vi "AllShipsSunk.vi"(0 "object in":refnum<class "Map.lvclass">, 5 "error in (no error)":errorcluster) -> (14 "object out":refnum<class "Map.lvclass">, 16 "AllShipsSunk?":bool, 19 "error out":errorcluster)   [LabVIEW 2015, in "Map.lvclass"]
doc: "Returns true if all ships on the map are sunk."
uses:
  Map.lvclass
  Map.lvclass/Map.ctl
  Battleship_class/Battleship.lvclass
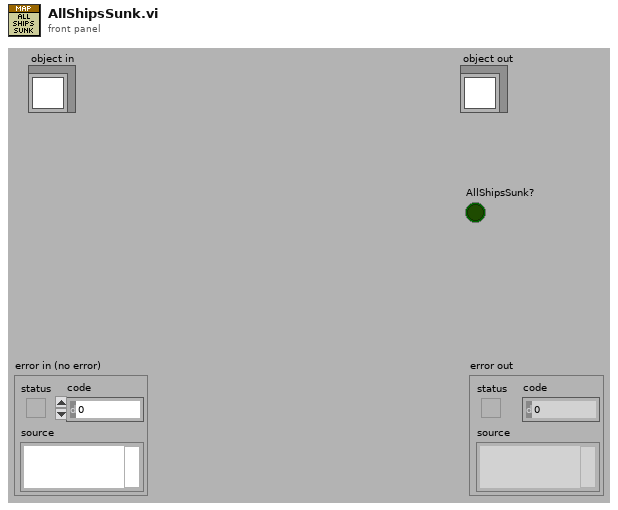
[diagram p1: front panel]
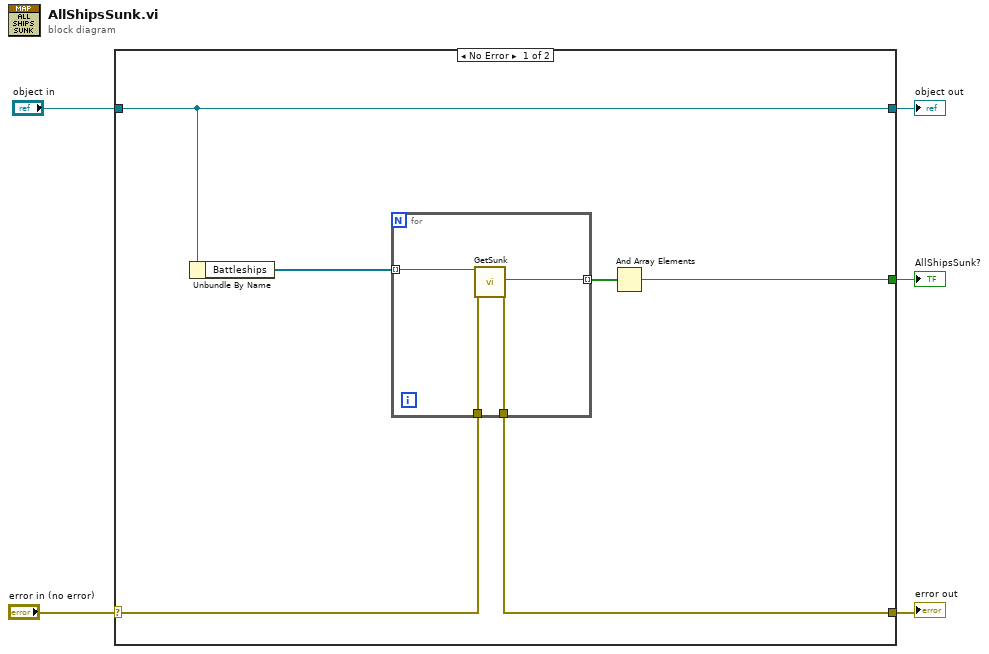
[diagram p0: block diagram]
diagram:
  n1 = case shown="No Error" "error in (no error)" {
    selector: "error in (no error)" -> [w9 w17]
    tunnel: [w8 w17] -> w4
    tunnel: [w11 w16] -> w2
    tunnel: "object in" -> [w11 w16]
    tunnel: [w6 _] -> w1
    frame No Error {
      n2 = Unbundle By Name(w11) -> ("Battleships"=w10:refnum<class "Battleship.lvclass">[])
      n3 = for {
        tunnel: w10 -> [w15] mode=indexing
        tunnel: w9 -> [w14]
        tunnel: [w13] -> w8
        tunnel: [w12] -> w7 mode=indexing
        n4 = call-dynamic "GetSunk.vi"("object in"=w15, "error in (no error)"=w14) -> ("Sunk?"=w12:bool, "error out"=w13:errorcluster)  [unwired: 15 in, 1 out]
      }
      n5 = And Array Elements(Boolean array=w7) -> (logical AND=w6:bool)
    }
    frame Error {
    }
  }
  "error out" <- w4
  "object out" <- w2
  "AllShipsSunk?" <- w1
